vi "Determine Sector Edge Location.vi"() -> (2 "Left Sector Edge":u8, 3 "Right Sector Edge":u8)   [LabVIEW 2013]
doc: "Takes the average sector intensities and compares each average to the threshold value to determine which sector the edge is located in."
uses:
  Globals/Accumulated Sector Intensity.vi
  Globals/Sector Parameter Global.vi
  <vilib>/rvi/FIFO/Fifo_Resource/nirvififoEmulationReadFpgaImpl.vi
  <vilib>/rvi/DataTransferAndStorage/Container/Common/niFpgaContainerGetUniqueNameForEmu.vi
  <vilib>/rvi/DataTransferAndStorage/Container/XNode/niFpgaContainer.xnode
  <vilib>/rvi/FIFO/Fifo_Resource/nirvififoEmulationRead.vi
  <vilib>/rvi/interface/RandomDataEmulation/nirviRandomDataFpgaReadWriteTemplate.vi
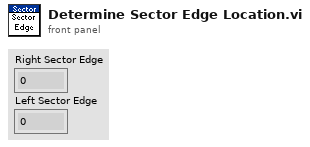
[diagram p1: front panel]
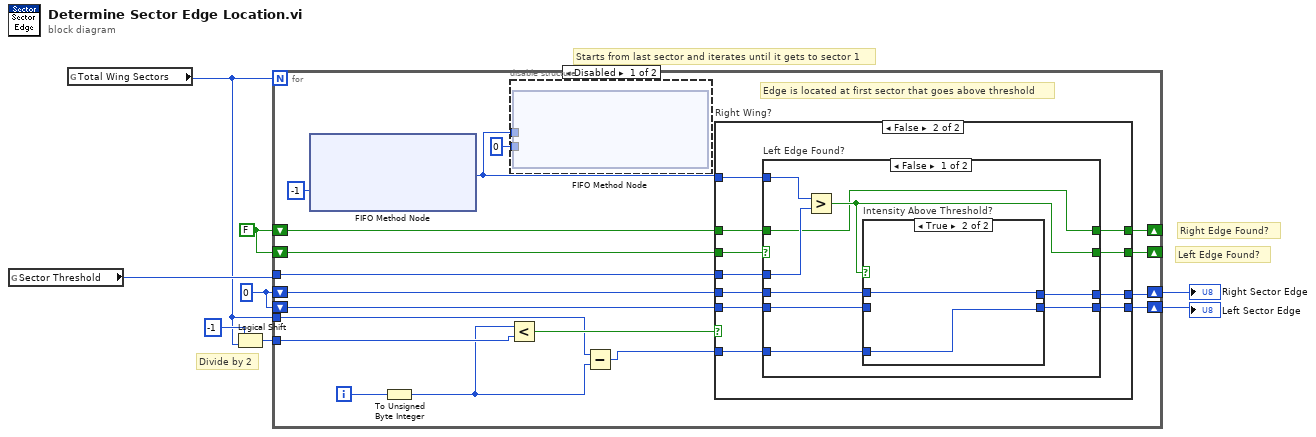
[diagram p0: block diagram]
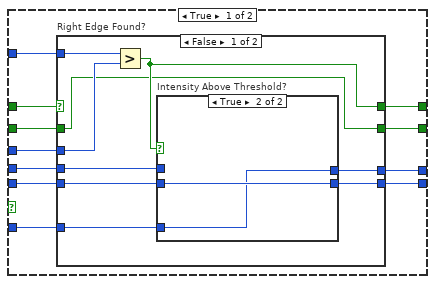
[diagram p3: hidden frame]
diagram:
  w3 = u8 0 ("Total Wing Sectors")
  w4 = FALSE ("Left Edge Found?")
  # "Starts from last sector and iterates until it gets to sector 1"
  # "Left Edge Found?"
  # "Right Edge Found?"
  # "Divide by 2"
  n1 = global read "Sector Parameter Global.vi" "Sector Threshold"() -> (w2:u8)
  n2 = global read "Accumulated Sector Intensity.vi" "Total Wing Sectors"() -> (w1:u8)
  n3 = Logical Shift(y=i16 -1, x=w1) -> (x << y=w5:u8)
  n4 = for {
    N: w1 -> [_]
    tunnel: w2 -> [w24]
    tunnel: w5 -> [w25]
    shift-right: [w22] -> _
    shift-left: w4 -> [w23]
    shift-right: [w15] -> _
    shift-left: w4 -> [w16]
    shift-right: [w20] -> w8
    shift-left: w3 -> [w19]
    shift-right: [w18] -> w7
    shift-left: w3 -> [w17]
    tunnel: w1 -> [w11]
    i -> [w21]
    # "Edge is located at first sector that goes above threshold"
    n5 = xnode ("FIFO Method Node")("Timeout"=-1) -> ("Element"=w14:u8)  [unwired: 1 in, 2 out]
    n6 = To Unsigned Byte Integer(number=w21) -> (unsigned 8bit integer=w10:u8)
    n7 = Less?(x=w10, y=w25) -> (x < y?=w26:bool)
    n8 = disable-structure shown="Disabled" {
      disable-tunnel: w14 -> [w28 _]
      disable-tunnel: 0 ("Timeout") -> [w27 _]
      frame Disabled {
        n9 = xnode ("FIFO Method Node")("Element"=w28, "Timeout"=w27) -> ()  [unwired: 1 in, 2 out]
      }
      frame Enabled {
      }
    }
    n10 = Subtract(x=w11, y=w10) -> (x-y=w9:u8)
    n11 = case "Right Wing?" shown="False" w26 {
      tunnel: w14 -> [w38 w67]
      tunnel: w24 -> [w37 w66]
      tunnel: w23 -> [w39 w58]
      tunnel: [w36 w65] -> w22
      tunnel: w9 -> [w35 w64]
      tunnel: [w34 w63] -> w20
      tunnel: w19 -> [w33 w62]
      tunnel: [w32 w61] -> w18
      tunnel: w17 -> [w31 w60]
      tunnel: w16 -> [w30 w59]
      tunnel: [w29 w57] -> w15
      frame True {
        n12 = case "Right Edge Found?" shown="False" w39 {
          selector: w39 -> [_ w53]
          tunnel: w38 -> [w48 _]
          tunnel: w37 -> [w47 _]
          tunnel: [w46 w53] -> w36
          tunnel: w35 -> [w45 _]
          tunnel: [w44 w56] -> w34
          tunnel: w33 -> [w43 w56]
          tunnel: [w42 w55] -> w32
          tunnel: w31 -> [w41 w55]
          tunnel: w30 -> [w40 w54]
          tunnel: [w40 w54] -> w29
          frame False {
            n13 = Greater?(x=w48, y=w47) -> (0:w46:bool)
            n14 = case "Intensity Above Threshold?" shown="True" w46 {
              tunnel: w45 -> [_ w51]
              tunnel: [w50 w51] -> w44
              tunnel: w43 -> [w50 _]
              tunnel: [w49 w52] -> w42
              tunnel: w41 -> [w49 w52]
              frame False {
              }
              frame True {
              }
            }
          }
          frame True {
          }
        }
      }
      frame False {
        n15 = case "Left Edge Found?" shown="False" w59 {
          selector: w59 -> [_ w81]
          tunnel: w67 -> [w76 _]
          tunnel: w66 -> [w75 _]
          tunnel: [w68 w82] -> w65
          tunnel: w64 -> [w74 _]
          tunnel: [w73 w84] -> w63
          tunnel: w62 -> [w72 w84]
          tunnel: [w71 w83] -> w61
          tunnel: w60 -> [w70 w83]
          tunnel: w58 -> [w68 w82]
          tunnel: [w69 w81] -> w57
          frame False {
            n16 = Greater?(x=w76, y=w75) -> (0:w69:bool)
            n17 = case "Intensity Above Threshold?" shown="True" w69 {
              tunnel: w74 -> [_ w79]
              tunnel: [w78 w80] -> w73
              tunnel: w72 -> [w78 w80]
              tunnel: [w77 w79] -> w71
              tunnel: w70 -> [w77 _]
              frame False {
              }
              frame True {
              }
            }
          }
          frame True {
          }
        }
      }
    }
  }
  "Right Sector Edge" <- w8
  "Left Sector Edge" <- w7
